vi "Send Stop Microgrid Msg.vi"(8 "error in":errorcluster, 10 "Data":variant, 11 "Remote Operation Abstract in":refnum<class "Remote Operation Abstract.lvclass">) -> (0 "error out":errorcluster, 3 "Remote Operation Abstract out":refnum<class "Remote Operation Abstract.lvclass">)   [LabVIEW 2018, in "Remote Operation Abstract.lvlib" / "Remote Operation Abstract.lvclass"]
uses:
  Remote Operation Abstract.lvclass
  C:/Program Files (x86)/National Instruments/LabVIEW 2018/vi.lib/ActorFramework/Actor/Actor.lvclass
  <vilib>/ActorFramework/Actor/Actor.lvclass/Actor.ctl
  Remote Operation Abstract.lvclass/Remote Operation Abstract.ctl
  Remote Operation Abstract Messages/Stop Microgrid Msg/Stop Microgrid Msg.lvclass/Stop Microgrid Msg.ctl
  <vilib>/ActorFramework/Message Enqueuer/Message Enqueuer.lvclass/Message Enqueuer.ctl
  <vilib>/ActorFramework/Message Enqueuer/Enqueue.vi
  Remote Operation Abstract Messages/Stop Microgrid Msg/Stop Microgrid Msg.lvclass
  C:/Program Files (x86)/National Instruments/LabVIEW 2018/vi.lib/ActorFramework/Message/Message.lvclass
  <vilib>/ActorFramework/Message Priority Queue/Priority Enqueue.vi
  <vilib>/ActorFramework/Actor/Actor.lvclass
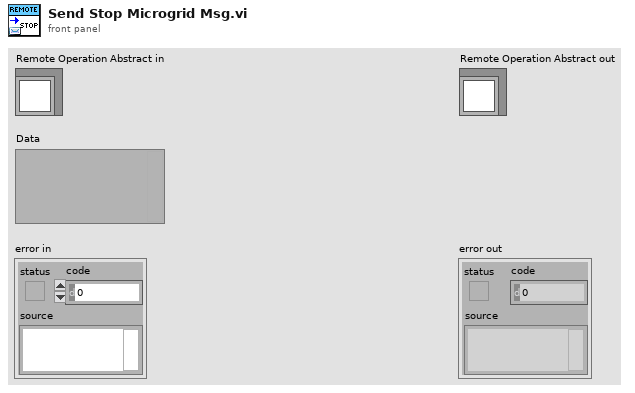
[diagram p1: front panel]
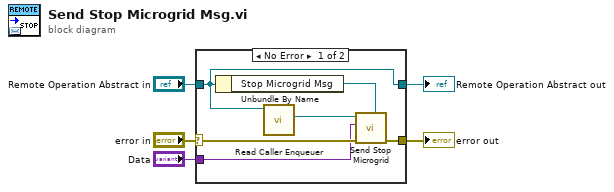
[diagram p0: block diagram]
diagram:
  n1 = case shown="No Error" "error in" {
    selector: "error in" -> [w10 w12]
    tunnel: [w6 w12] -> w4
    tunnel: [w11 w13] -> w2
    tunnel: "Remote Operation Abstract in" -> [w11 w13]
    tunnel: "Data" -> [w9 _]
    frame No Error {
      n2 = Unbundle By Name(w11) -> ("Stop Microgrid Msg"=w7:refnum<class "Stop Microgrid Msg.lvclass">)
      n3 = call <vilib>:"Read Caller Enqueuer.vi"("Actor"=w11) -> ("Caller Enqueuer"=w8:refnum<class "Message Enqueuer.lvclass">)  [unwired: 10 in]
      n4 = call "Send Stop Microgrid.vi"("Message Type"=w7, "error in (no error)"=w10, "Variant"=w9, "Message Enqueuer"=w8) -> ("error out"=w6:errorcluster)  [unwired: 6 in, 1 out]
    }
    frame Error {
    }
  }
  "error out" <- w4
  "Remote Operation Abstract out" <- w2
